vi "Instrument_Input.vi"() -> ()   [LabVIEW 2020]
doc: "This VI gets in commands from user as SOURce and MEASure and the calls a subVI to write and get the values from the file to return and also logs this event with time"
panel:
  out "Log file error":errorcluster
  out "Response":string
  in  "Command":string
  # "This VI give commands from user to another VI to store the data and then \nretrives it based on the command input"
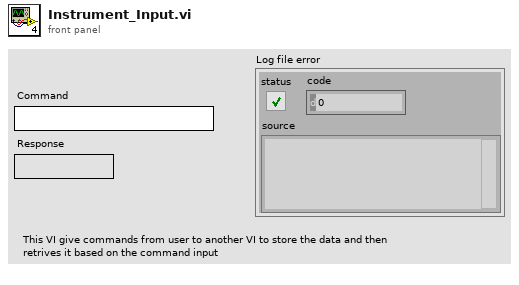
[diagram p1: front panel]
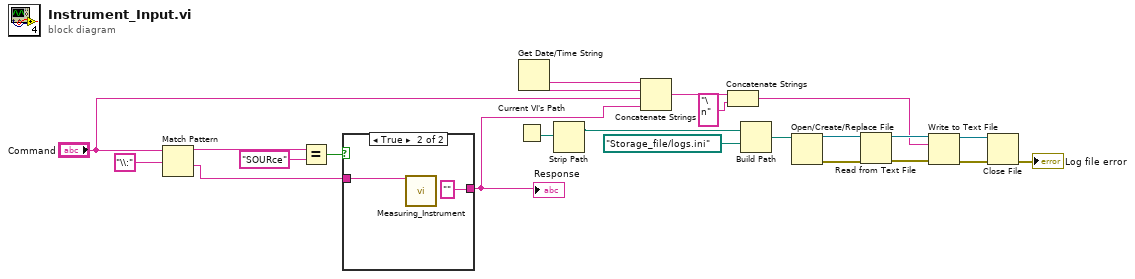
[diagram p0: block diagram]
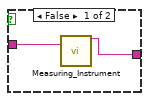
[diagram p2: hidden frame]
diagram:
  n1 = Match Pattern(string="Command", regular expression="\\:") -> (before substring=w22:string, after substring=w19:string)  [unwired: 1 in, 2 out]
  n2 = Equal?(x=w22, y="SOURce") -> (x = y?=w20:bool)
  n3 = case shown="True" w20 {
    tunnel: w19 -> [w25 w27]
    tunnel: [w24 "" ("String 3")] -> w10
    frame False {
      n4 = call "Measuring_Instrument.vi"("Read String"=w25) -> ("Readed Data"=w24:string)  [unwired: 14 in]
    }
    frame True, Default {
      n5 = call "Measuring_Instrument.vi"("Write String"=w27) -> ()  [unwired: 14 in, 1 out]
    }
  }
  "Response" <- w10
  n6 = Current VI's Path() -> (path=w16:path)
  n7 = Get Date/Time String() -> (date string=w13:string, time string=w12:string)  [unwired: 3 in]
  n8 = Strip Path(path=w16) -> (stripped path=w8:path)  [unwired: 1 out]
  n9 = Concatenate Strings(w13, w12, "Command", w10) -> (w3:string)
  n10 = Concatenate Strings(w3, "\n" ("string")) -> (w1:string)
  n11 = Build Path(base path=w8, name or relative path=path "Storage_file/logs.ini") -> (appended path=w14:path)
  n12 = Open/Create/Replace File(file path (use dialog)=w14) -> (refnum out=w5:refnum<file>, error out=w7:errorcluster)  [unwired: 5 in, 1 out]
  n13 = Read from Text File(file (use dialog)=w5, error in=w7) -> (refnum out=w4:refnum<file>, error out=w6:errorcluster)  [unwired: 2 in, 2 out]
  n14 = Write to Text File(file (use dialog)=w4, text=w1, error in=w6) -> (refnum out=w17:refnum<file>, error out=w18:errorcluster)  [unwired: 1 in, 1 out]
  n15 = Close File(refnum=w17, error in=w18) -> (error out=→"Log file error":errorcluster)  [unwired: 1 out]
